vi "Dipose Kinect.vi"(8 "error in (no error)":errorcluster, 11 "Kinect Session in":refnum<class "Kinect Session.lvclass">) -> (0 "error out":errorcluster)   [LabVIEW 2014, in "Kinect Library.lvlib"]
doc: "This function cleans up all of the Kinect sensor references and stops the Kinect. Although it is not strictly required to call this function before ending VI Execution, it will prevent memory leaking which may eventually require LabVIEW to be restarted."
uses:
  Kinect Library.lvlib
  Kinect Session Class/Kinect Session.lvclass
  Microsoft.Kinect
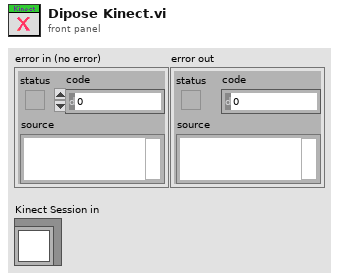
[diagram p1: front panel]
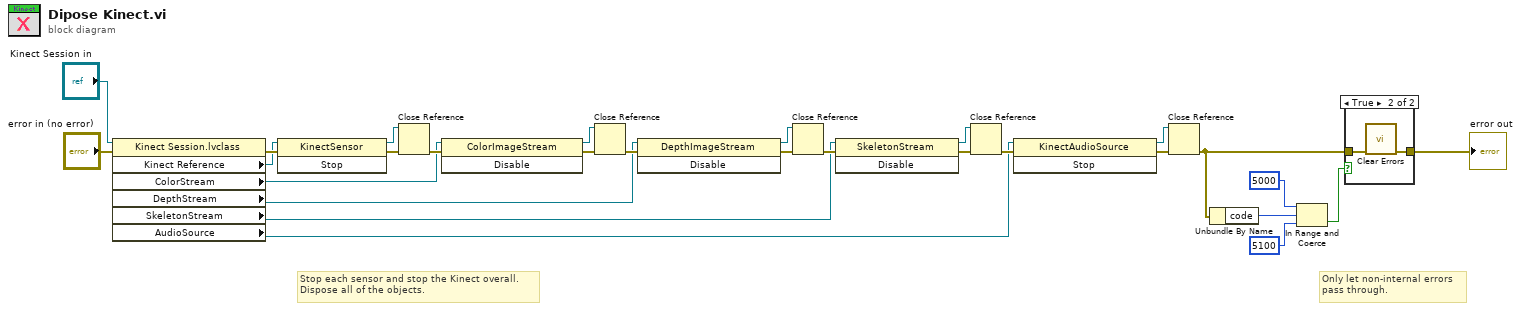
[diagram p0: block diagram]
diagram:
  # "Only let non-internal errors\npass through."
  # "Stop each sensor and stop the Kinect overall. \nDispose all of the objects."
  n1 = property class="Kinect Session.lvclass"(reference="Kinect Session in", error in="error in (no error)") -> (error out=w26:errorcluster, "Kinect Reference"=w11:refnum<k24>, "ColorStream"=w10:refnum<k24>, "DepthStream"=w9:refnum<k24>, "SkeletonStream"=w8:refnum<k24>, "AudioSource"=w7:refnum<k24>)  [unwired: 1 out]
  n2 = invoke class="KinectSensor" method="Stop"(reference=w11, error in=w26) -> (reference out=w27:refnum<k24>, error out=w25:errorcluster)  [unwired: 1 in, 1 out]
  n3 = Close Reference(reference=w27, error in (no error)=w25) -> (error out=w24:errorcluster)
  n4 = invoke class="ColorImageStream" method="Disable"(reference=w10, error in=w24) -> (reference out=w23:refnum<k24>, error out=w22:errorcluster)  [unwired: 1 in, 1 out]
  n5 = Close Reference(reference=w23, error in (no error)=w22) -> (error out=w21:errorcluster)
  n6 = invoke class="DepthImageStream" method="Disable"(reference=w9, error in=w21) -> (reference out=w20:refnum<k24>, error out=w19:errorcluster)  [unwired: 1 in, 1 out]
  n7 = Close Reference(reference=w20, error in (no error)=w19) -> (error out=w18:errorcluster)
  n8 = invoke class="SkeletonStream" method="Disable"(reference=w8, error in=w18) -> (reference out=w17:refnum<k24>, error out=w16:errorcluster)  [unwired: 1 in, 1 out]
  n9 = Close Reference(reference=w17, error in (no error)=w16) -> (error out=w15:errorcluster)
  n10 = invoke class="KinectAudioSource" method="Stop"(reference=w7, error in=w15) -> (reference out=w14:refnum<k24>, error out=w13:errorcluster)  [unwired: 1 in, 1 out]
  n11 = Close Reference(reference=w14, error in (no error)=w13) -> (error out=w3:errorcluster)
  n12 = Unbundle By Name(w3) -> ("code"=w6:i32)
  n13 = In Range and Coerce(upper limit=5000, x=w6, lower limit=5100) -> (In Range?=w2:bool)  [unwired: 1 out]
  n14 = case shown="True" w2 {
    tunnel: w3 -> [w29 w31]
    tunnel: [w29 w30] -> w1
    frame False {
    }
    frame True {
      n15 = call <vilib>:"Clear Errors.vi"("error in (no error)"=w31) -> ("error out"=w30:errorcluster)  [unwired: 5 in, 1 out]
    }
  }
  "error out" <- w1
